vi "PostControlPanelRefnum.vi"(8 "error in (no error)":errorcluster, 9 "VI Refnum":refnum<vi>, 10 "Panel":string, 11 "GRMActor in":refnum<class "GRMActor.lvclass">) -> (0 "error out":errorcluster, 3 "GRMActor out":refnum<class "GRMActor.lvclass">)   [LabVIEW 2020, in "GRMActor.lvlib" / "GRMActor.lvclass"]
uses:
  GRMActor.lvclass
  C:/Program Files/National Instruments/LabVIEW 2020/vi.lib/ActorFramework/Actor/Actor.lvclass
  <vilib>/ActorFramework/Actor/Actor.lvclass/Actor.ctl
  Interface/DockStation Messages/InsertDevicePanel Msg/InsertDevicePanel Msg.lvclass/InsertDevicePanel Msg.ctl
  <vilib>/ActorFramework/Message Enqueuer/Message Enqueuer.lvclass/Message Enqueuer.ctl
  <vilib>/ActorFramework/Message Enqueuer/Enqueue.vi
  Interface/DockStation Messages/InsertDevicePanel Msg/InsertDevicePanel Msg.lvclass
  C:/Program Files/National Instruments/LabVIEW 2020/vi.lib/ActorFramework/Message/Message.lvclass
  <vilib>/ActorFramework/Message Priority Queue/Priority Enqueue.vi
  <vilib>/ActorFramework/Actor/Actor.lvclass
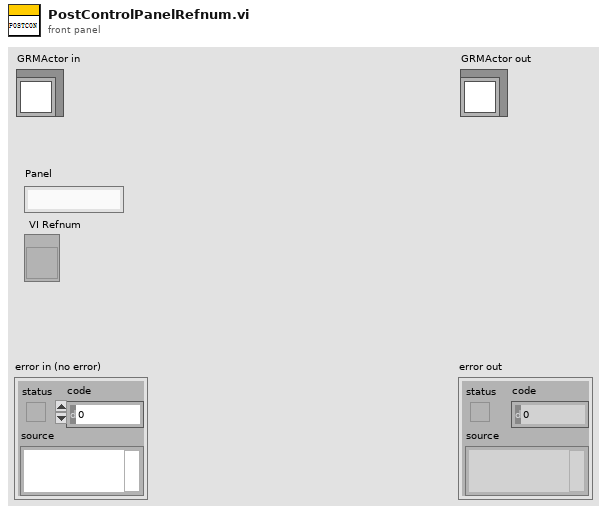
[diagram p1: front panel]
types:
  T1 = enum32{"Invalid", "Standard", "Closed", "Hidden", "Minimized", "Maximized"}
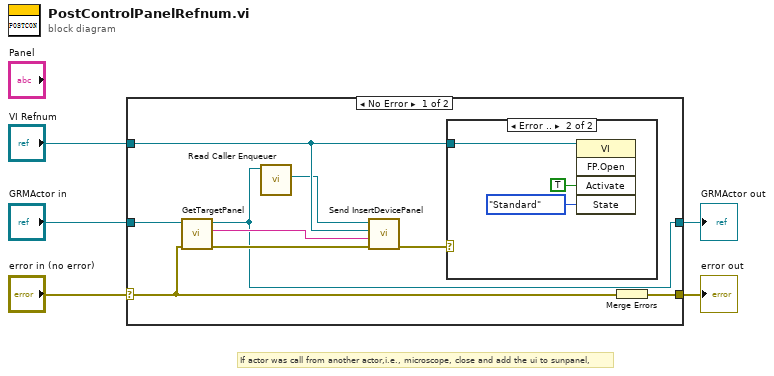
[diagram p0: block diagram]
diagram:
  # "If actor was call from another actor,i.e., microscope, close and add the ui to sunpanel,"
  n1 = case shown="No Error" "error in (no error)" {
    selector: "error in (no error)" -> [w11 w19]
    tunnel: [w14 w19] -> w4
    tunnel: [w6 w18] -> w3
    tunnel: "GRMActor in" -> [w12 w18]
    tunnel: "VI Refnum" -> [w13 _]
    frame No Error {
      n2 = call-dynamic "GetTargetPanel.vi"("error in (no error)"=w11, "GRMActor in"=w12) -> ("error out"=w10:errorcluster, "TargetPanel"=w7:string, "GRMActor out"=w6:refnum<class "GRMActor.lvclass">)  [unwired: 7 in]
      n3 = call <vilib>:"Read Caller Enqueuer.vi"("Actor"=w6) -> ("Caller Enqueuer"=w9:refnum<class "Message Enqueuer.lvclass">)  [unwired: 10 in]
      n4 = call "Send InsertDevicePanel.vi"("error in (no error)"=w10, "Panel"=w7, "VI Refnum"=w13, "Message Enqueuer"=w9) -> ("error out"=w8:errorcluster)  [unwired: 6 in, 1 out]
      n5 = case shown="Error .." w8 {
        tunnel: w13 -> [_ w17]
        frame No Error {
        }
        frame Error {
          n6 = invoke class="VI" method="FP.Open"(reference=w17, "Activate"=TRUE ("Activate?"), "State"=T1."Standard") -> ()  [unwired: 2 in, 5 out]
        }
      }
      n7 = Merge Errors(w11) -> (w14:errorcluster)
    }
    frame Error {
    }
  }
  "error out" <- w4
  "GRMActor out" <- w3
